vi "ErrorDefinitionSQLite_TestClass.vi"() -> ()   [LabVIEW 2018]
uses:
  <userlib>/_express/ErrorDefinitionSQLite/ErrorContent.ctl
  <userlib>/_express/ErrorDefinitionSQLite/ErrorDefinitionSQLite.lvclass
panel:
  out "Errors":T1
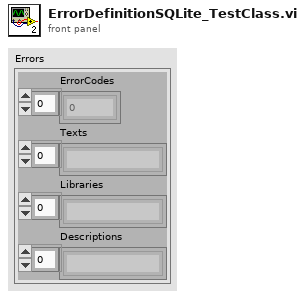
[diagram p1: front panel]
types:
  T1 = typedef "ErrorDefinitionSQLite.lvclass/ErrorContent.ctl" = cluster{"ErrorCodes":i32[], "Texts":string[], "Libraries":string[], "Descriptions":string[]}
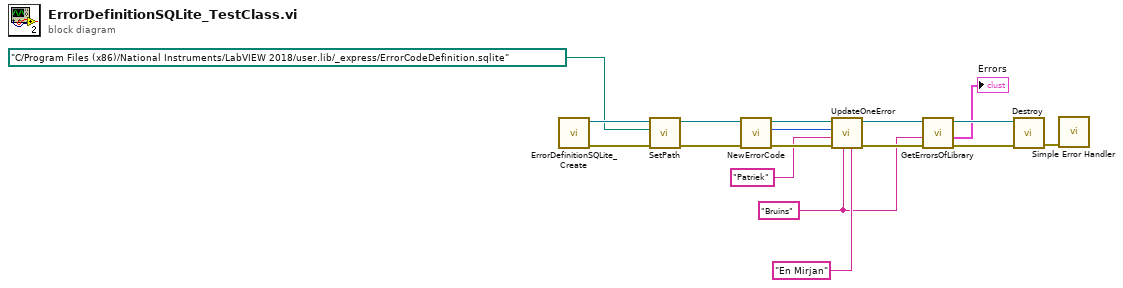
[diagram p0: block diagram]
diagram:
  w3 = "Bruins" ("Library")
  n1 = call <userlib>:"ErrorDefinitionSQLite_Create.vi"() -> ("ErrorOut"=w16:errorcluster, "Reference out"=w17:refnum<class "ErrorDefinitionSQLite.lvclass">)  [unwired: 10 in]
  n2 = call-dynamic "SetPath.vi"("ErrorIn"=w16, "Path"=path "C:/Program Files (x86)/National Instruments/LabVIEW 2018/user.lib/_express/ErrorCodeDefinition.sqlite", "ReferenceIn"=w17) -> ("ErrorOut"=w14:errorcluster, "ReferenceOut"=w15:refnum<class "ErrorDefinitionSQLite.lvclass">)  [unwired: 7 in]
  n3 = call-dynamic "NewErrorCode.vi"("ErrorIn"=w14, "ReferenceIn"=w15) -> ("ErrorOut"=w12:errorcluster, "NewErrorCode"=w6:i32, "ReferenceOut"=w13:refnum<class "ErrorDefinitionSQLite.lvclass">)  [unwired: 7 in]
  n4 = call-dynamic "UpdateOneError.vi"("Description"="En Mirjan", "Library"=w3, "ErrorIn"=w12, "Text"="Patriek", "ErrorCode"=w6, "ReferenceIn"=w13) -> ("ErrorOut"=w10:errorcluster, "ReferenceOut"=w11:refnum<class "ErrorDefinitionSQLite.lvclass">)  [unwired: 4 in]
  n5 = call-dynamic "GetErrorsOfLibrary.vi"("ErrorIn"=w10, "LibraryName"=w3, "ReferenceIn"=w11) -> ("ErrorOut"=w8:errorcluster, "Errors"=→"Errors":T1, "ReferenceOut"=w9:refnum<class "ErrorDefinitionSQLite.lvclass">)  [unwired: 6 in]
  n6 = call-dynamic "Destroy.vi"("ErrorIn"=w8, "Reference in"=w9) -> ("ErrorOut"=w1:errorcluster)  [unwired: 8 in, 1 out]
  n7 = call <vilib>:"Simple Error Handler.vi"("error in (no error)"=w1) -> ()  [unwired: 4 in, 5 out]
